vi "Start Sync.vi"(8 "error in (no error)":errorcluster, 11 "gRPC Server in":refnum<class "MeasurementService.lvclass">) -> (0 "error out":errorcluster, 3 "gRPC Server out":refnum<class "MeasurementService.lvclass">)   [LabVIEW 2020, in "MeasurementLink Measurement Server.lvlib" / "MeasurementService.lvclass"]
uses:
  MeasurementService.lvclass
  \\nyduscanal\measurement-services-labview/Source/Measurement Service Template_lv/MeasurementLink Measurement Server Internal/RPC Service/MeasurementService/MeasurementService.lvclass
  MeasurementLink Measurement Server Internal/RPC Service/MeasurementService/MeasurementService.lvclass/MeasurementService.ctl
  MeasurementLink Measurement Template/Measurement Results.ctl
  MeasurementLink Measurement Server Internal/RPC Messages/ni_measurementlink_measurement_v1_GetMetadataResponse.ctl
  MeasurementLink Measurement Server Internal/RPC Messages/ni_measurementlink_measurement_v1_MeasurementDetails.ctl
  MeasurementLink Measurement Server Internal/RPC Messages/ni_measurementlink_measurement_v1_MeasurementSignature.ctl
  MeasurementLink Measurement Server Internal/RPC Messages/ni_measurementlink_measurement_v1_ConfigurationParameter.ctl
  MeasurementLink Measurement Server Internal/RPC Messages/ni_measurementlink_measurement_v1_ConfigurationParameter_AnnotationsEntry.ctl
  MeasurementLink Measurement Server Internal/RPC Messages/google_protobuf_Any.ctl
  MeasurementLink Measurement Server Internal/RPC Messages/ni_measurementlink_measurement_v1_Output.ctl
  MeasurementLink Measurement Server Internal/RPC Messages/ni_measurementlink_measurement_v1_UserInterfaceDetails.ctl
  415e3662-0215-4442-959e-9b67fb8742ba.vi
  <vilib>/gRPC/LabVIEW gRPC Library/Server API/Translate Protobuf Error.vi
  <vilib>/AdvancedString/1D String Array to Delimited String.vi
  <vilib>/gRPC/LabVIEW gRPC Library/Server API/Server/Get Server DLL Path.vi
  MeasurementService.lvclass/MeasurementService.ctl
  MeasurementLink Measurement Server Internal/RPC Service/MeasurementService/MeasurementService.lvclass
  MeasurementLink Measurement Server.lvlib
  MeasurementLink Measurement Template/MeasurementLink Measurement Template.lvlib
  MeasurementLink Measurement Server Internal/MeasurementLink Measurement Server Internal.lvlib
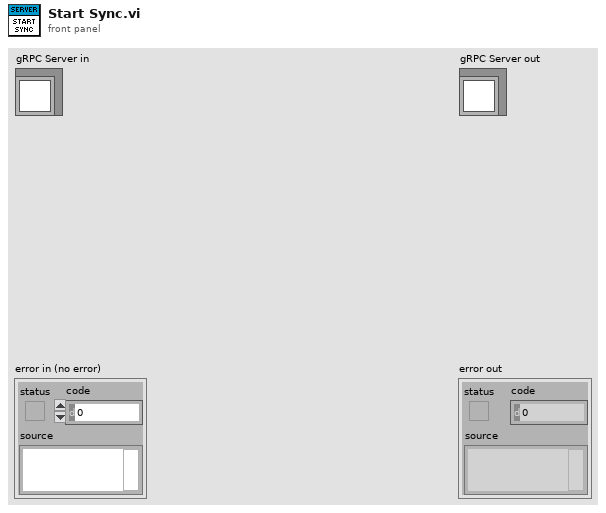
[diagram p1: front panel]
types:
  T1 = typedef "MeasurementLink Measurement Server Internal.lvlib/ni_measurementlink_measurement_v1_MeasurementSignature.ctl" = cluster{"configuration_parameters_message_type":string, "configuration_parameters":T2[], "configuration_defaults":T4, "outputs_message_type":string, "outputs":T5[]}
  T2 = typedef "MeasurementLink Measurement Server Internal.lvlib/ni_measurementlink_measurement_v1_ConfigurationParameter.ctl" = cluster{"field_number":i32, "type":i32, "name":string, "repeated":bool, "annotations":T3[]}
  T3 = typedef "MeasurementLink Measurement Server Internal.lvlib/ni_measurementlink_measurement_v1_ConfigurationParameter_AnnotationsEntry.ctl" = cluster{"key":string, "value":string}
  T4 = typedef "MeasurementLink Measurement Server Internal.lvlib/google_protobuf_Any.ctl" = cluster{"type_url":string, "value":u8[]}
  T5 = typedef "MeasurementLink Measurement Server Internal.lvlib/ni_measurementlink_measurement_v1_Output.ctl" = cluster{"field_number":i32, "type":i32, "name":string, "repeated":bool}
  T6 = typedef "MeasurementLink Measurement Server Internal.lvlib/ni_measurementlink_measurement_v1_GetMetadataResponse.ctl" = cluster{"measurement_details":T7, "measurement_signature":T1, "user_interface_details":T8[]}
  T7 = typedef "MeasurementLink Measurement Server Internal.lvlib/ni_measurementlink_measurement_v1_MeasurementDetails.ctl" = cluster{"display_name":string, "version":string}
  T8 = typedef "MeasurementLink Measurement Server Internal.lvlib/ni_measurementlink_measurement_v1_UserInterfaceDetails.ctl" = cluster{"file_url":string}
  T9 = typedef "MeasurementLink Measurement Server Internal.lvlib/MeasurementService.lvclass/Server Internal UEs.ctl" = cluster{"MeasurementService GetMetadata Internal UE":refnum<user-event>, "MeasurementService Measure Internal UE":refnum<user-event>}
  T10 = typedef "MeasurementLink Measurement Server Internal.lvlib/MeasurementService.lvclass/Server gRPC UEs.ctl" = cluster{"MeasurementService GetMetadata gRPC UE":refnum<user-event>, "MeasurementService Measure gRPC UE":refnum<user-event>}
  T11 = typedef "MeasurementLink Measurement Template.lvlib/Measurement Results.ctl" = cluster{"Array out":dbl[]}
  T12 = typedef "grpc-lvsupport-release.lvlib/grpcId.ctl" = u64
  T13 = typedef "MeasurementLink Measurement Template.lvlib/Measurement Configuration.ctl" = cluster{"Array in":dbl[]}
  T14 = typedef "grpc-lvsupport-release.lvlib/Any.ctl" = cluster{"Type Url":string, "Bytes":u8[]}
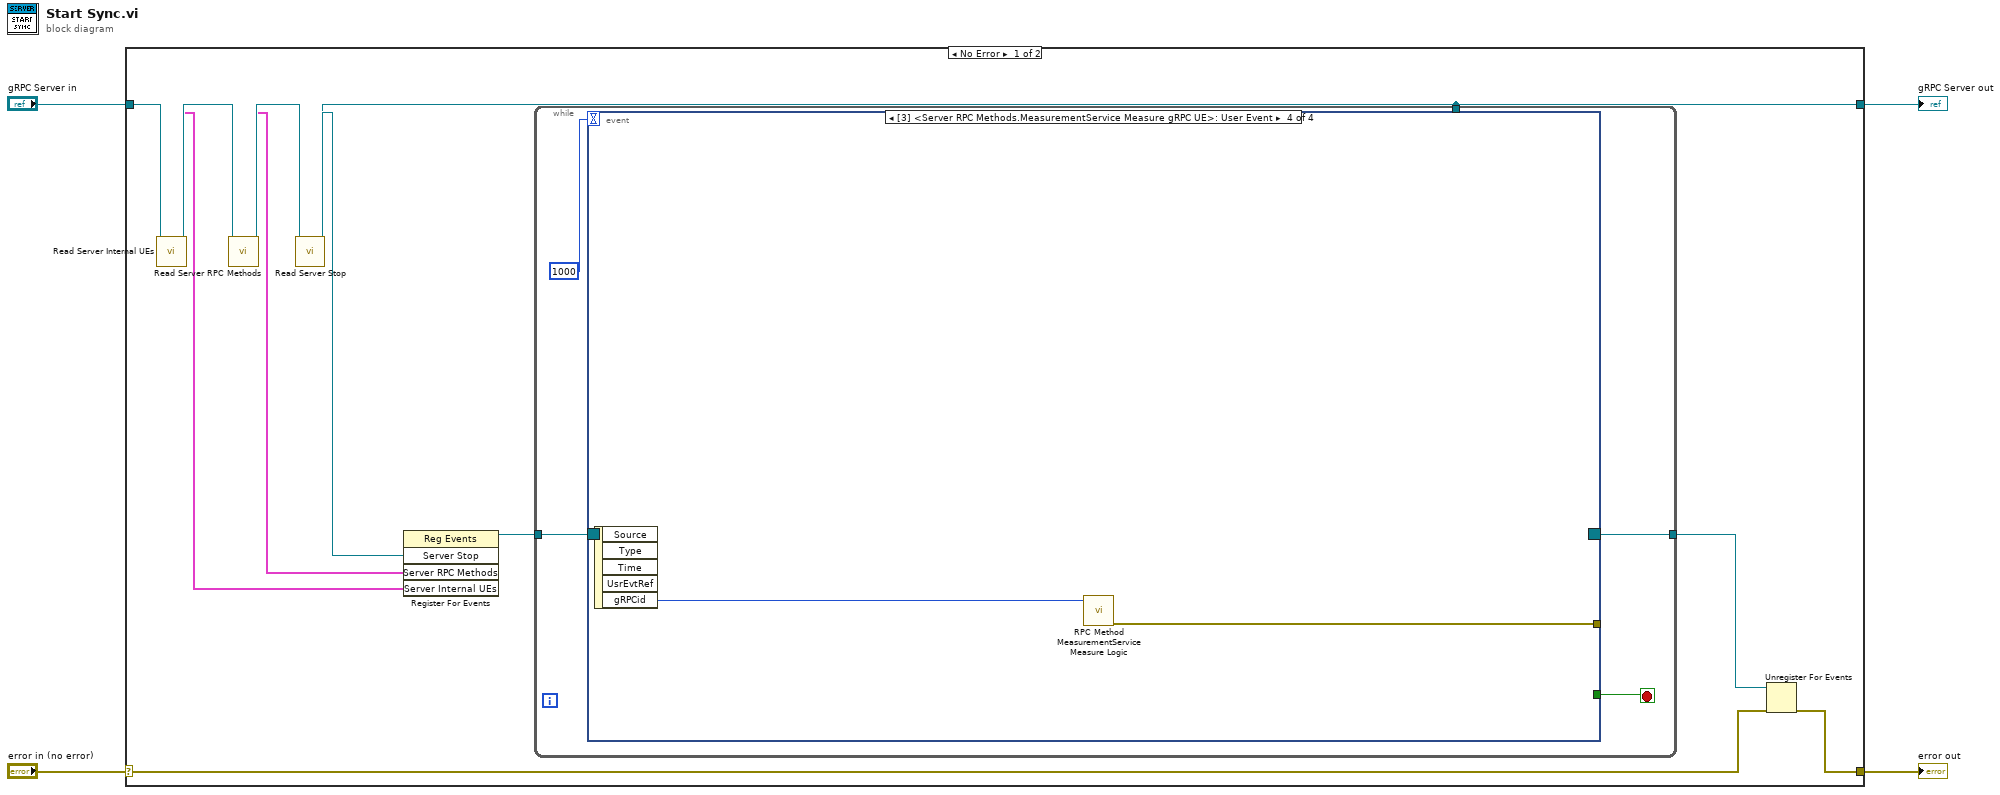
[diagram p0: block diagram]
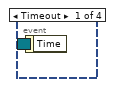
[diagram p2: hidden frame]
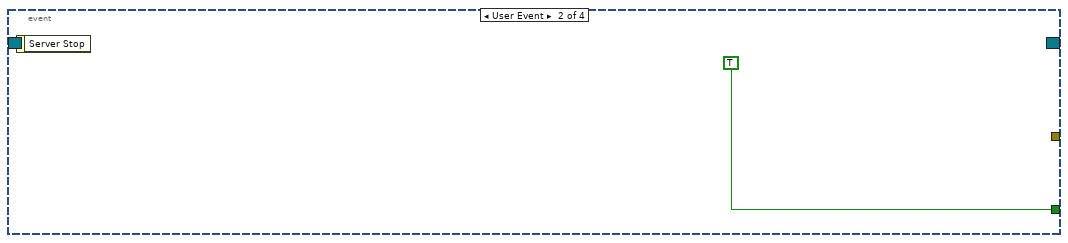
[diagram p3: hidden frame]
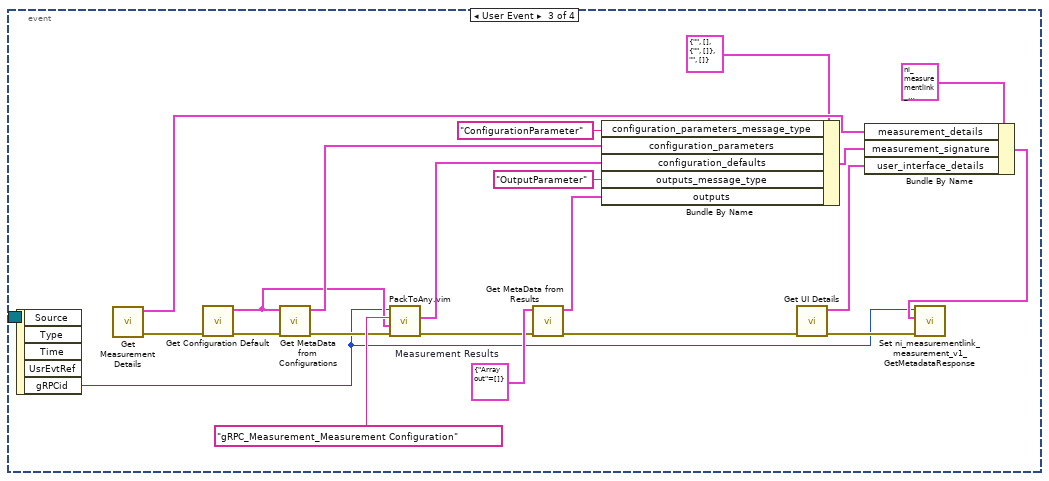
[diagram p4: hidden frame]
diagram:
  n1 = case shown="No Error" "error in (no error)" {
    selector: "error in (no error)" -> [w9 w45]
    tunnel: [w8 w45] -> w3
    tunnel: [w5 w44] -> w1
    tunnel: "gRPC Server in" -> [w15 w44]
    frame No Error {
      n2 = call "Read Server Internal UEs.vi"("SignalGeneratorService in"=w15) -> ("Server Internal UEs"=w13:T9, "SignalGeneratorService out"=w14:refnum<class "MeasurementService.lvclass">)  [unwired: 8 in, 1 out]
      n3 = call "Read Server RPC Methods.vi"("SignalGeneratorService in"=w14) -> ("Server RPC Methods"=w7:T10, "SignalGeneratorService out"=w12:refnum<class "MeasurementService.lvclass">)  [unwired: 8 in, 1 out]
      n4 = call-dynamic "Read Server Stop.vi"("iService in"=w12) -> ("Server Stop"=w6:refnum<user-event>, "iService out"=w5:refnum<class "MeasurementService.lvclass">)  [unwired: 8 in, 1 out]
      n5 = register-events(w6, w7, w13) -> (reference out=w11:refnum<event-registration>)  [unwired: 2 in, 1 out]
      n6 = while {
        tunnel: w11 -> [w19]
        tunnel: [w17] -> w10
        tunnel: w5 -> [_]
        stop <- w18 stop-if-true
        n7 = event "RPC Methods Event Structure" shown="[3] <Server RPC Methods.MeasurementService Measure gRPC UE>: User Event" {
          selector: w19 -> [_ _ _ _]
          dyn-events: [_ _ _ _] -> w17
          timeout: 1000 -> [_ _ _ _]
          tunnel: [_ TRUE _ _] -> w18
          tunnel: [_ _ _ w42] -> _
          event Timeout {
            n8 = event-data() -> ()  [unwired: 1 in, 1 out]
          }
          event User Event {
            n9 = event-data() -> ()  [unwired: 1 in, 1 out]
          }
          event User Event {
            w39 = T11 {"Array out"=[]}  # Measurement Results
            n10 = event-data() -> ("gRPCid"=w25:T12)  [unwired: 1 in, 4 out]
            n11 = call "Get Measurement Details.vi"() -> ("error out"=w31:errorcluster, "Measurement Details"=w22:T7)  [unwired: 9 in, 1 out]
            n12 = call "Get Configuration Default.vi"("error in (no error)"=w31) -> ("error out"=w30:errorcluster, "Measurement Configuration Default"=w29:T13)  [unwired: 9 in]
            n13 = call "Get MetaData from Configurations.vi"("error in"=w30, "Configuration Cluster"=w29) -> ("error out"=w35:errorcluster, "configuration_parameters"=w41:T2[])  [unwired: 8 in]
            n14 = call "PackToAny.vim"("error in"=w35, "Data To Pack"=w29, "Message Type"="gRPC_Measurement_Measurement Configuration", "gRPCid in"=w25) -> ("error out"=w34:errorcluster, "Any"=w33:T14)  [unwired: 5 in, 1 out]
            n15 = call "Get MetaData from Results.vi"("error in"=w34, "Configuration Cluster"=w39) -> ("error out"=w32:errorcluster, "outputs"=w40:T5[])  [unwired: 8 in]
            n16 = Bundle By Name(cluster=T1 {"configuration_parameters_message_type"="", "configuration_parameters"=[], "configuration_defaults"={"type_url"="", "value"=[]}, "outputs_message_type"="", "outputs"=[]} ("ni_measurements_v1_MeasurementSignature"), "configuration_parameters_message_type"="ConfigurationParameter" ("configuration_parameters_messagetype"), "configuration_parameters"=w41, "configuration_defaults"=w33, "outputs_message_type"="OutputParameter" ("configuration_parameters_messagetype"), "outputs"=w40) -> (w23:T1)
            n17 = call "Get UI Details.vi"("error in"=w32) -> ("error out"=w27:errorcluster, "user_interface_details"=w24:T8[])  [unwired: 9 in]
            n18 = Bundle By Name(cluster=T6 {"measurement_details"={"display_name"="", "version"=""}, "measurement_signature"={"configuration_parameters_message_type"="", "configuration_parameters"=[], "configuration_defaults"={"type_url"="", "value"=[]}, "outputs_message_type"="", "outputs"=[]}, "user_interface_details"=[]} ("package_templatemessage"), "measurement_details"=w22, "measurement_signature"=w23, "user_interface_details"=w24) -> (w26:T6)
            n19 = call "Set ni_measurementlink_measurement_v1_GetMetadataResponse.vi"("error in (no error)"=w27, "package_templatemessage"=w26, "gRPCid"=w25) -> ()  [unwired: 8 in, 1 out]
          }
          event User Event {
            n20 = event-data() -> ("gRPCid"=w43:T12)  [unwired: 1 in, 4 out]
            n21 = call "RPC Method MeasurementService Measure Logic.vi"("gRPCid in"=w43) -> ("error out"=w42:errorcluster)  [unwired: 10 in]
          }
        }
      }
      n22 = Unregister For Events(event registration refnum=w10, error in=w9) -> (error out=w8:errorcluster)
    }
    frame Error {
    }
  }
  "error out" <- w3
  "gRPC Server out" <- w1
